vi "Set Font.vi"(8 "error in (no error)":errorcluster, 9 "Text formatting":T1={"Font"="Arial", "Size"=18.0, "Italic"=FALSE, "Bold"=FALSE, "Underline"=FALSE, "Color"=0}, 10 "Shape refnum":refnum<k7>) -> (0 "error out":errorcluster, 2 "Shape refnum out":refnum<k7>)   [LabVIEW 2020, in "lvpptx.lvlib"]
uses:
  lvpptx.lvlib
  Font.ctl
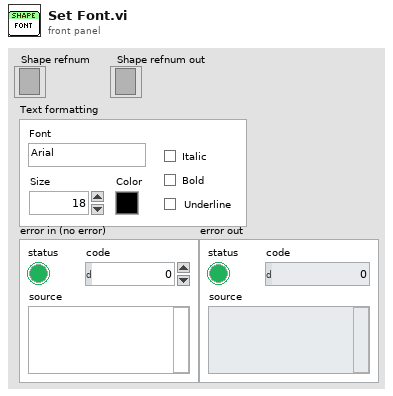
[diagram p1: front panel]
types:
  T1 = typedef "lvpptx.lvlib/Font.ctl" = cluster{"Font":string, "Size":dbl, "Italic":bool, "Bold":bool, "Underline":bool, "Color":u32}
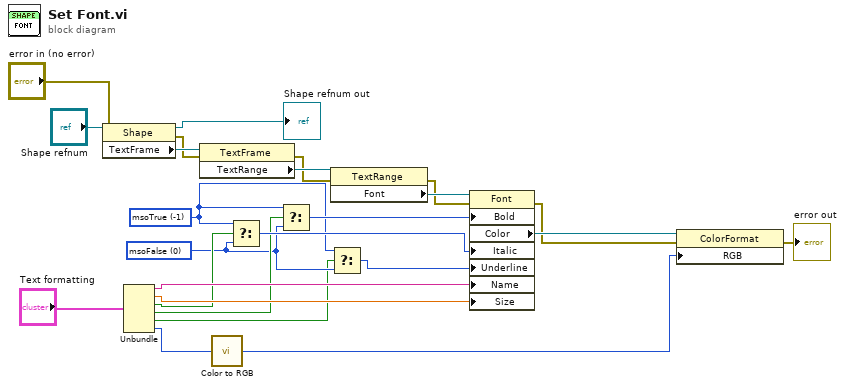
[diagram p0: block diagram]
diagram:
  w14 = 0 items=["msoTrue"=-1, "msoFalse"=0, "msoCTrue"=1, "msoTriStateToggle"=-3, "msoTriStateMixed"=-2] ("Bold")
  w13 = -1 items=["msoTrue"=-1, "msoFalse"=0, "msoCTrue"=1, "msoTriStateToggle"=-3, "msoTriStateMixed"=-2] ("Bold")
  n1 = property class="Shape"(reference="Shape refnum", error in="error in (no error)") -> (reference out=→"Shape refnum out":refnum<k7>, error out=w7:errorcluster, "TextFrame"=w25:refnum<k7>)
  n2 = Unbundle("Text formatting") -> ("Font"=w22:string, "Size"=w21:dbl, "Italic"=w19:bool, "Bold"=w17:bool, "Underline"=w12:bool, "Color"=w6:u32)
  n3 = property class="TextFrame"(reference=w25, error in=w7) -> (error out=w8:errorcluster, "TextRange"=w24:refnum<k7>)  [unwired: 1 out]
  n4 = call "Color to RGB.vi"("Color"=w6) -> ("32bit out"=w5:u32)  [unwired: 4 in]
  n5 = Select(t=w13, s=w19, f=w14) -> (s? t:f=w18:i32)
  n6 = Select(t=w13, s=w17, f=w14) -> (s? t:f=w16:i32)
  n7 = property class="TextRange"(reference=w24, error in=w8) -> (error out=w9:errorcluster, "Font"=w23:refnum<k7>)  [unwired: 1 out]
  n8 = Select(t=w13, s=w12, f=w14) -> (s? t:f=w15:i32)
  n9 = property class="Font"(reference=w23, error in=w9, "Bold"=w16, "Italic"=w18, "Underline"=w15, "Name"=w22, "Size"=w21) -> (error out=w10:errorcluster, "Color"=w20:refnum<k7>)  [unwired: 1 out]
  n10 = property class="ColorFormat"(reference=w20, error in=w10, "RGB"=w5) -> (error out=→"error out":errorcluster)  [unwired: 1 out]
